vi "SubVI_ResAcc.vi"(2 "속도":dbl=100000.0, 3 "샘플 개수":i32=2000, 4 "timeout (s)":dbl=10.0 caption="타임아웃(초)" format="%0.2f", 5 "error in":errorcluster caption="에러 입력", 7 "stop (T)":bool=TRUE caption="정지(T)") -> (14 "task out":refnum<k21> caption="태스크 출력", 15 "data":dynamicdata(graph) caption="데이터", 19 "error out":errorcluster caption="에러 출력")   [LabVIEW 2013]
doc: "NI-DAQmx를 사용하여 태스크를 생성, 편집, 실행합니다. NI-DAQmx가 지원하는 디바이스의 완전한 리스트는 NI-DAQ Readme를 참조하십시오.\n\n이 익스프레스 VI를 블록다이어그램에 놓으면 DAQ 어시스턴트가 시작되어 새로운 태스크를 생성합니다, 태스크를 생성한 후, DAQ 어시스턴트 익스프레스 VI를 더블 클릭하여 해당 태스크를 편집할 수 있습니다. 연속적인 측정 또는 생성을 위해서는 DAQ 어시스턴트 익스프레스 주위에 while 루프를 놓습니다.\n\n연속적인 단일 포인트 입력 또는 출력의 경우 DAQ 어시스턴트 익스프레스 VI는 최적의 성능을 제공하지 않을 수도 있습니다. 높은 성능을 가진 단일 포인트 I/O 어플리케이션을 생성하는 기술에 대한 예제는 examples\\DAQmx\\Analog In\\Measure Voltage.llb의 Cont Acq&Graph Voltage-Single Point Optimization VI를 참조하십시오."
uses:
  <vilib>/DAQmx/read.llb/DAQmx Read.vi
  <vilib>/DAQmx/read.llb/DAQmx Read (Analog 1D Wfm NChan NSamp).vi
  <vilib>/DAQmx/create/channels.llb/DAQmx Create Channel (TEDS-AI-Voltage-Basic).vi
  <vilib>/DAQmx/create/channels.llb/DAQmx Create Channel (AI-Voltage-Basic).vi
  <vilib>/DAQmx/configure/timing.llb/DAQmx Timing (Sample Clock).vi
  <vilib>/DAQmx/configure/trigger.llb/DAQmx Trigger.vi
  <vilib>/DAQmx/configure/trigger.llb/DAQmx Start Trigger (Digital Edge).vi
  <vilib>/DAQmx/miscellaneous.llb/DAQmx Fill In Error Info.vi
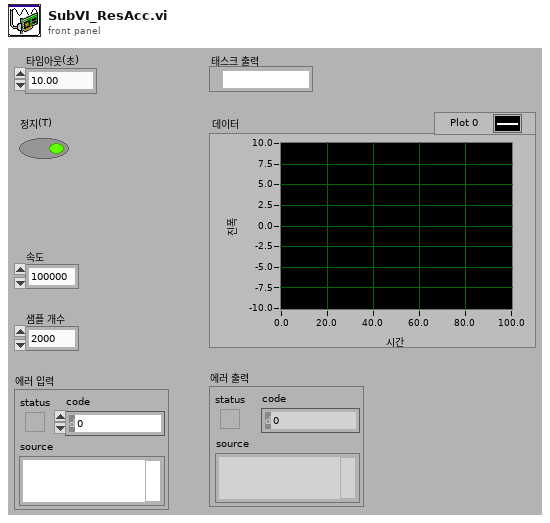
[diagram p1: front panel]
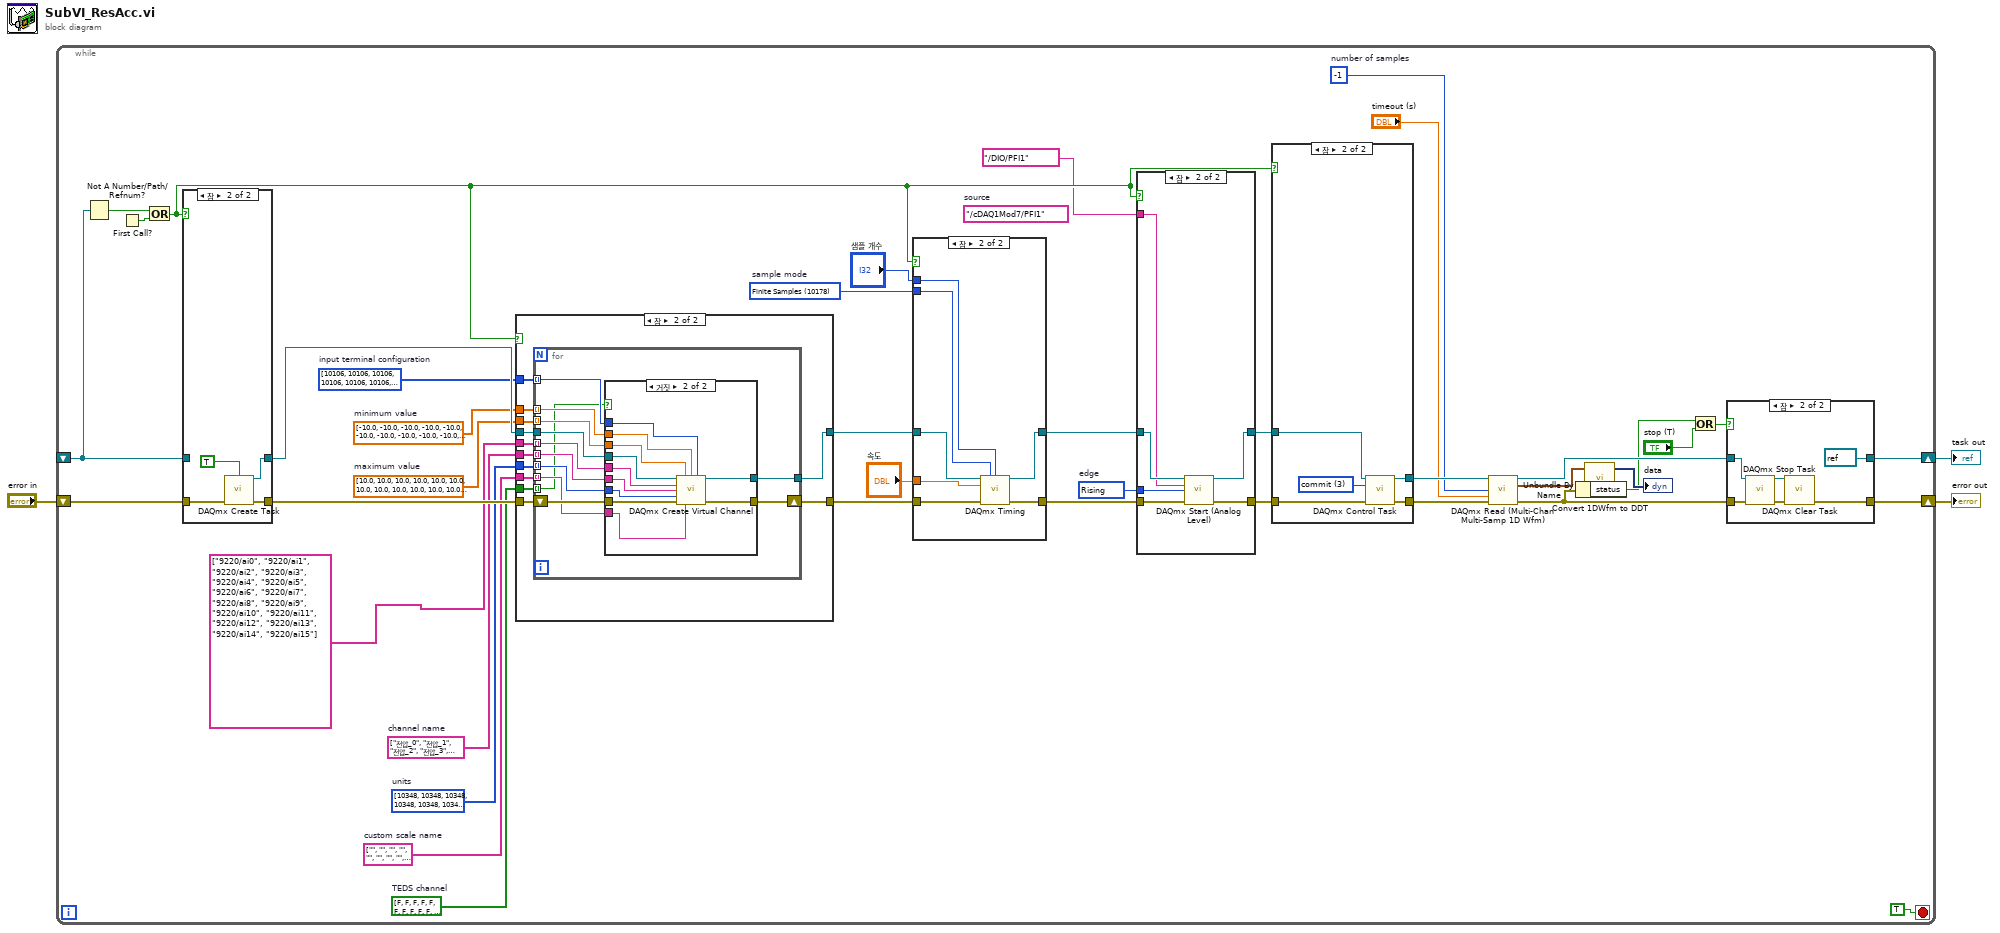
[diagram p0: block diagram]
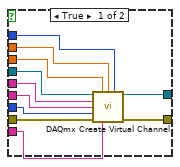
[diagram p7: hidden frame]
diagram:
  n1 = while {
    shift-right: [w11] -> w1
    shift-left: _ -> [w40]
    shift-right: [w9] -> w2
    shift-left: "error in" -> [w41]
    stop <- TRUE stop-if-true
    w15 = -1  # number of samples
    w21 = 10280 items=["Rising"=10280, "Falling"=10171]  # edge
    (unwired) "/cDAQ1Mod7/PFI1"  # source
    w24 = 10178 items=["Finite Samples"=10178, "Continuous Samples"=10123, "Hardware Timed Single Point"=12522]  # sample mode
    w29 = bool[] [FALSE, FALSE, FALSE, FALSE, FALSE, FALSE, FALSE, FALSE, FALSE, FALSE, FALSE, FALSE, FALSE, FALSE, FALSE, FALSE]  # TEDS channel
    w30 = string[] ["", "", "", "", "", "", "", "", "", "", "", "", "", "", "", ""]  # custom scale name
    w31 = i32[] [10348, 10348, 10348, 10348, 10348, 10348, 10348, 10348, 10348, 10348, 10348, 10348, 10348, 10348, 10348, 10348] items=["Volts"=10348, "From TEDS"=12516, "From Custom Scale"=10065]  # units
    w32 = string[] ["전압_0", "전압_1", "전압_2", "전압_3", "전압_4", "전압_5", "전압_6", "전압_7", "전압_8", "전압_9", "전압_10", "전압_11", "전압_12", "전압_13", "전압_14", "전압_15"]  # channel name
    w34 = dbl[] [10.0, 10.0, 10.0, 10.0, 10.0, 10.0, 10.0, 10.0, 10.0, 10.0, 10.0, 10.0, 10.0, 10.0, 10.0, 10.0]  # maximum value
    w35 = dbl[] [-10.0, -10.0, -10.0, -10.0, -10.0, -10.0, -10.0, -10.0, -10.0, -10.0, -10.0, -10.0, -10.0, -10.0, -10.0, -10.0]  # minimum value
    w36 = i32[] [10106, 10106, 10106, 10106, 10106, 10106, 10106, 10106, 10106, 10106, 10106, 10106, 10106, 10106, 10106, 10106] items=["default"=-1, "RSE"=10083, "NRSE"=10078, "Differential"=10106, "Pseudodifferential"=12529]  # input terminal configuration
    n2 = Not A Number/Path/Refnum?(number/path/refnum=w40) -> (NaN/Path/Refnum?=w39:bool)
    n3 = First Call?() -> (First Call?: T/F=w42:bool)
    n4 = Or(x=w39, y=w42) -> (x .or. y?=w20:bool)
    n5 = case "케이스 구조" shown="참" w20 {
      tunnel: [w125 w129] -> w38
      tunnel: w40 -> [w125 _]
      tunnel: [w124 w128] -> w37
      tunnel: w41 -> [w124 w126]
      frame False {
      }
      frame True {
        n6 = call <vilib>:"DAQmx Create Task.vi"("auto cleanup"=TRUE, "error in"=w126) -> ("task out"=w129:refnum<k21>, "error out"=w128:errorcluster)  [unwired: 12 in]
      }
    }
    n7 = case "케이스 구조" shown="참" w20 {
      tunnel: [w77 w87] -> w28
      tunnel: w38 -> [w77 w89]
      tunnel: [w76 w86] -> w27
      tunnel: w37 -> [w76 w88]
      tunnel: w36 -> [_ w85]
      tunnel: w35 -> [_ w84]
      tunnel: w34 -> [_ w83]
      tunnel: tag[] ["9220/ai0", "9220/ai1", "9220/ai2", "9220/ai3", "9220/ai4", "9220/ai5", "9220/ai6", "9220/ai7", "9220/ai8", "9220/ai9", "9220/ai10", "9220/ai11", "9220/ai12", "9220/ai13", "9220/ai14", "9220/ai15"] -> [_ w82]
      tunnel: w32 -> [_ w81]
      tunnel: w31 -> [_ w80]
      tunnel: w30 -> [_ w79]
      tunnel: w29 -> [_ w78]
      frame False {
      }
      frame True {
        n8 = for "For 루프" {
          tunnel: w89 -> [w101]
          tunnel: [w99] -> w87
          tunnel: w85 -> [w97] mode=indexing
          tunnel: w84 -> [w96] mode=indexing
          tunnel: w83 -> [w95] mode=indexing
          tunnel: w82 -> [w94] mode=indexing
          tunnel: w81 -> [w93] mode=indexing
          tunnel: w80 -> [w92] mode=indexing
          tunnel: w79 -> [w91] mode=indexing
          shift-right: [w98] -> w86
          shift-left: w88 -> [w100]
          tunnel: w78 -> [w90] mode=indexing
          n9 = case "케이스 구조" shown="거짓" w90 {
            tunnel: w101 -> [w112 w123]
            tunnel: w100 -> [w111 w122]
            tunnel: [w110 w121] -> w99
            tunnel: [w109 w120] -> w98
            tunnel: w97 -> [w108 w119]
            tunnel: w96 -> [w107 w118]
            tunnel: w95 -> [w106 w117]
            tunnel: w94 -> [w105 w116]
            tunnel: w93 -> [w104 w115]
            tunnel: w92 -> [w103 w114]
            tunnel: w91 -> [w102 w113]
            frame True {
              n10 = call-poly <vilib>:"DAQmx Create Virtual Channel.vi"("task in"=w112, "maximum value"=w106, "minimum value"=w107, "input terminal configuration"=w108, "physical channels"=w105, "name to assign"=w104, "units"=w103, "error in"=w111, "custom scale name"=w102) -> ("task out"=w110:refnum<k21>, "error out"=w109:errorcluster)  [unwired: 5 in]
            }
            frame False {
              n11 = call-poly <vilib>:"DAQmx Create Virtual Channel.vi"("task in"=w123, "maximum value"=w117, "minimum value"=w118, "input terminal configuration"=w119, "physical channels"=w116, "name to assign"=w115, "units"=w114, "error in"=w122, "custom scale name"=w113) -> ("task out"=w121:refnum<k21>, "error out"=w120:errorcluster)  [unwired: 5 in]
            }
          }
        }
      }
    }
    n12 = case "케이스 구조" shown="참" w20 {
      tunnel: [w68 w70] -> w23
      tunnel: w28 -> [w68 w73]
      tunnel: [w67 w69] -> w22
      tunnel: w27 -> [w67 w71]
      tunnel: "샘플 개수" -> [_ w75]
      tunnel: w24 -> [_ w74]
      tunnel: "속도" -> [_ w72]
      frame False {
      }
      frame True {
        n13 = call-poly <vilib>:"DAQmx Timing.vi"("task/channels in"=w73, "sample mode"=w74, "samples per channel"=w75, "rate"=w72, "error in"=w71) -> ("task out"=w70:refnum<k21>, "error out"=w69:errorcluster)  [unwired: 9 in]
      }
    }
    n14 = case "케이스 구조" shown="참" w20 {
      tunnel: [w60 w64] -> w19
      tunnel: w23 -> [w60 w66]
      tunnel: [w59 w63] -> w18
      tunnel: w22 -> [w59 w65]
      tunnel: tag "/DIO/PFI1" ("source") -> [_ w62]
      tunnel: w21 -> [_ w61]
      frame False {
      }
      frame True {
        n15 = call-poly "DAQmx Start (Analog Level).vi"("task/channels in"=w66, "source"=w62, "edge"=w61, "error in"=w65) -> ("task out"=w64:refnum<k21>, "error out"=w63:errorcluster)  [unwired: 10 in]
      }
    }
    n16 = case "케이스 구조" shown="참" w20 {
      tunnel: [w53 w57] -> w17
      tunnel: w19 -> [w53 w58]
      tunnel: [w52 w55] -> w16
      tunnel: w18 -> [w52 w56]
      frame False {
      }
      frame True {
        w54 = 3 items=["verify"=2, "reserve"=4, "commit"=3, "unreserve"=5, "abort"=6] ("action")
        n17 = call <vilib>:"DAQmx Control Task.vi"("task/channels in"=w58, "action"=w54, "error in"=w56) -> ("task out"=w57:refnum<k21>, "error out"=w55:errorcluster)  [unwired: 11 in]
      }
    }
    n18 = call-poly "DAQmx Read (Multi-Chan Multi-Samp 1D Wfm).vi"("task/channels in"=w17, "number of samples per channel"=w15, "timeout"="timeout (s)", "error in"=w16) -> ("task out"=w10:refnum<k21>, "data"=w14:waveform(dbl)[], "error out"=w8:errorcluster)  [unwired: 9 in]
    n19 = Unbundle By Name(w8) -> ("status"=w7:bool)
    n20 = call <vilib>:"Convert 1DWfm to DDT.vi"("Array of Waveforms"=w14) -> ("Dynamic Data Type"=→"data":dynamicdata)  [unwired: 3 in]
    n21 = Or(x=w7, y="stop (T)") -> (x .or. y?=w5:bool)
    n22 = case "케이스 구조" shown="참" w5 {
      tunnel: [w45 refnum<k21> refnum ("task in")] -> w11
      tunnel: w10 -> [w45 w51]
      tunnel: [w44 w48] -> w9
      tunnel: w8 -> [w44 w50]
      frame False {
      }
      frame True {
        n23 = call <vilib>:"DAQmx Stop Task.vi"("task/channels in"=w51, "error in"=w50) -> ("task out"=w47:refnum<k21>, "error out"=w49:errorcluster)  [unwired: 12 in]
        n24 = call <vilib>:"DAQmx Clear Task.vi"("task in"=w47, "error in"=w49) -> ("error out"=w48:errorcluster)  [unwired: 13 in]
      }
    }
  }
  "error out" <- w2
  "task out" <- w1
